vi "MS SQL_Read_Global_Date_v2.vi"(6 "index":i32, 7 "Audit":T1, 8 "error in (no error)":errorcluster, 11 "Ref in":T2={"MS SQL Connection"=refnum, "UDL File"=path "", "Time"="", "DCODE"="", "WIP+1"=0, "MC No?"=0, "POKAYOKE?"=FALSE, "Expected Result"="", "Result [Status]"="", "Clock"=0.0, "RFID"="", "WIP Queue"=refnum, "TS Parameter"={"ProfitCenterCode"="", "LineCode"="", "WorkOrderNumber"="", "Model"="", "Model_with_Prefix"="", "VendorCode"="", "SetParameterDateCode"="", "PokaYoke"=0, "Target"=1, "Live_DateCode"="", "CustomerPartNumber"="", "Hand"="", "Ent_Stamp"=timestamp(0 s since 1904-01-01), "sBarcode"=FALSE, "FCA"=0, "STS_CD"=0.0}, "Data_Queue"=[], "RFID Serial No."=""} {"TS Parameter"."FCA" format="%01d"; "TS Parameter"."Target" min=1 max=100000; "TS Parameter"."PokaYoke" min=0 max=1}) -> (0 "error out":errorcluster, 2 "Date":string[](array[string]), 3 "Ref Out":T2={"MS SQL Connection"=refnum, "UDL File"=path "", "Time"="", "DCODE"="", "WIP+1"=0, "MC No?"=0, "POKAYOKE?"=FALSE, "Expected Result"="", "Result [Status]"="", "Clock"=0.0, "RFID"="", "WIP Queue"=refnum, "TS Parameter"={"ProfitCenterCode"="", "LineCode"="", "WorkOrderNumber"="", "Model"="", "Model_with_Prefix"="", "VendorCode"="", "SetParameterDateCode"="", "PokaYoke"=0, "Target"=1, "Live_DateCode"="", "CustomerPartNumber"="", "Hand"="", "Ent_Stamp"=timestamp(0 s since 1904-01-01), "sBarcode"=FALSE, "FCA"=0, "STS_CD"=0.0}, "Data_Queue"=[], "RFID Serial No."=""} {"TS Parameter"."FCA" format="%01d"; "TS Parameter"."Target" min=1 max=100000; "TS Parameter"."PokaYoke" min=0 max=1})   [LabVIEW 2020]
uses:
  Controls/TD SQL.ctl
  <vilib>/addons/database/Connection.llb/Conn ObjectReference.ctl
  Controls/WIP_State.ctl
  Controls/TS_Parameter.ctl
  <menus>/Controls/Devaseelan Style/ONOFF Small.ctl
  <vilib>/addons/database/Connection.llb/Conn Execute.vi
  <vilib>/addons/database/Recordset.llb/Rec Fetch Recordset Data (R).vi
  <vilib>/addons/database/Recordset.llb/Rec Destroy - Connection.vi
  <userlib>/_OpenG.lib/array/array.llb/Remove Duplicates from 1D Array (String)__ogtk.vi
  <vilib>/addons/database/NI_Database_API.lvlib
panel:
  out "array w/ subset deleted":string[](array[string])
  out "concatenated string":string
  out "result string":string
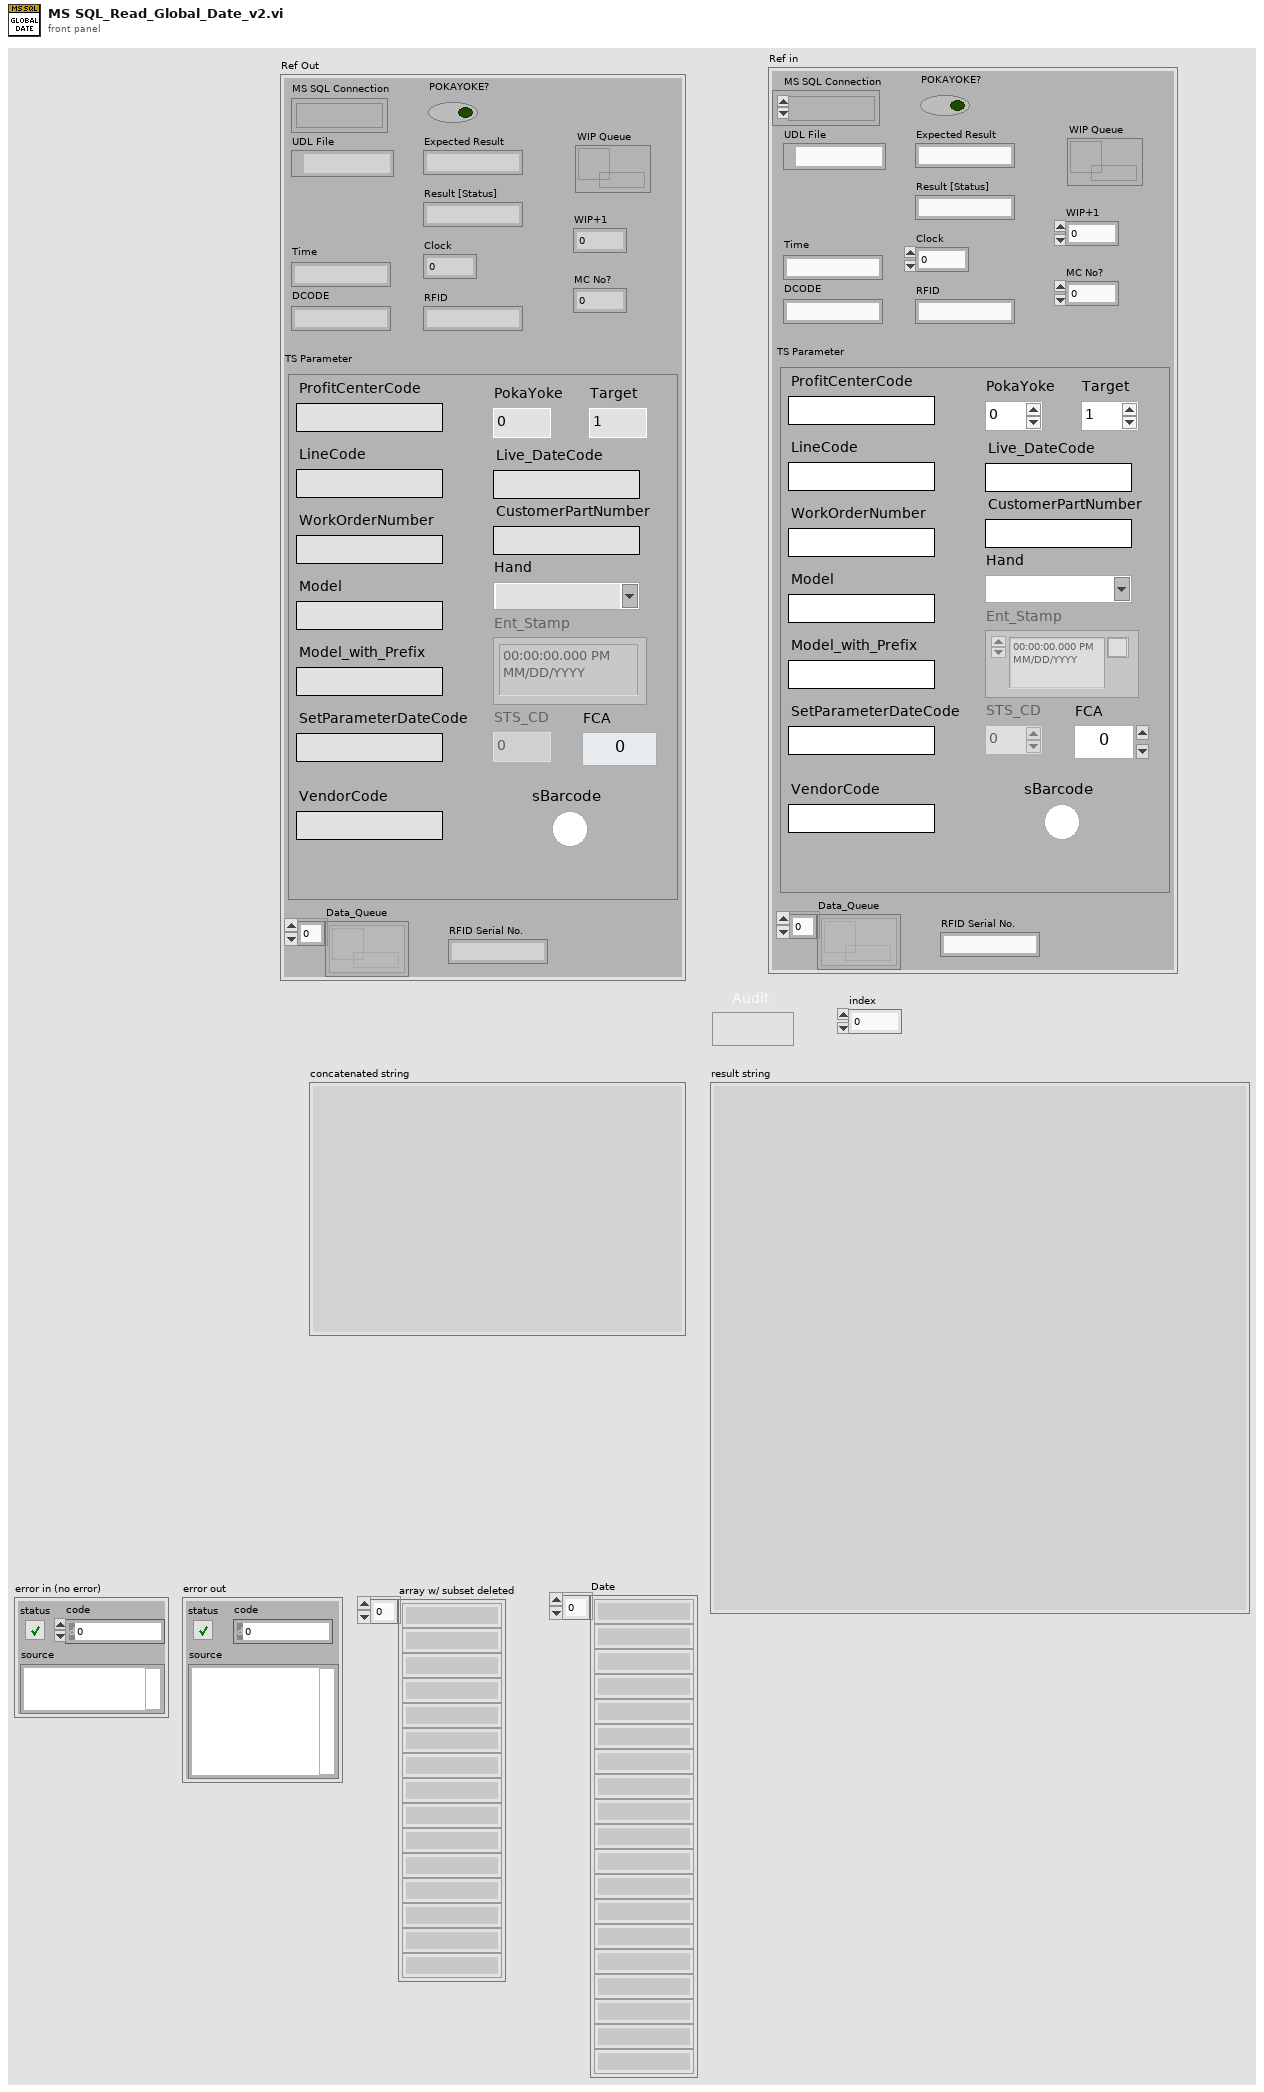
[diagram p1: front panel]
types:
  T1 = typedef "ONOFF Small.ctl" = bool
  T2 = typedef "TD SQL.ctl" = cluster{"MS SQL Connection":T3, "UDL File":path, "Time":string, "DCODE":string, "WIP+1":i64, "MC No?":i32, "POKAYOKE?":bool, "Expected Result":string, "Result [Status]":string, "Clock":dbl, "RFID":string, "WIP Queue":refnum<queue>, "TS Parameter":T4, "Data_Queue":refnum<queue>[], "RFID Serial No.":string}
  T3 = typedef "NI_Database_API.lvlib/Conn ObjectReference.ctl" = refnum<k1>
  T4 = typedef "TS_Parameter.ctl" = cluster{"ProfitCenterCode":string, "LineCode":string, "WorkOrderNumber":string, "Model":string, "Model_with_Prefix":string, "VendorCode":string, "SetParameterDateCode":string, "PokaYoke":i32, "Target":i32, "Live_DateCode":string, "CustomerPartNumber":string, "Hand":string, "Ent_Stamp":timestamp, "sBarcode":bool, "FCA":i32, "STS_CD":dbl}
  T5 = typedef "NI_Database_API.lvlib/Rec ObjectReference.ctl" = refnum<k1>
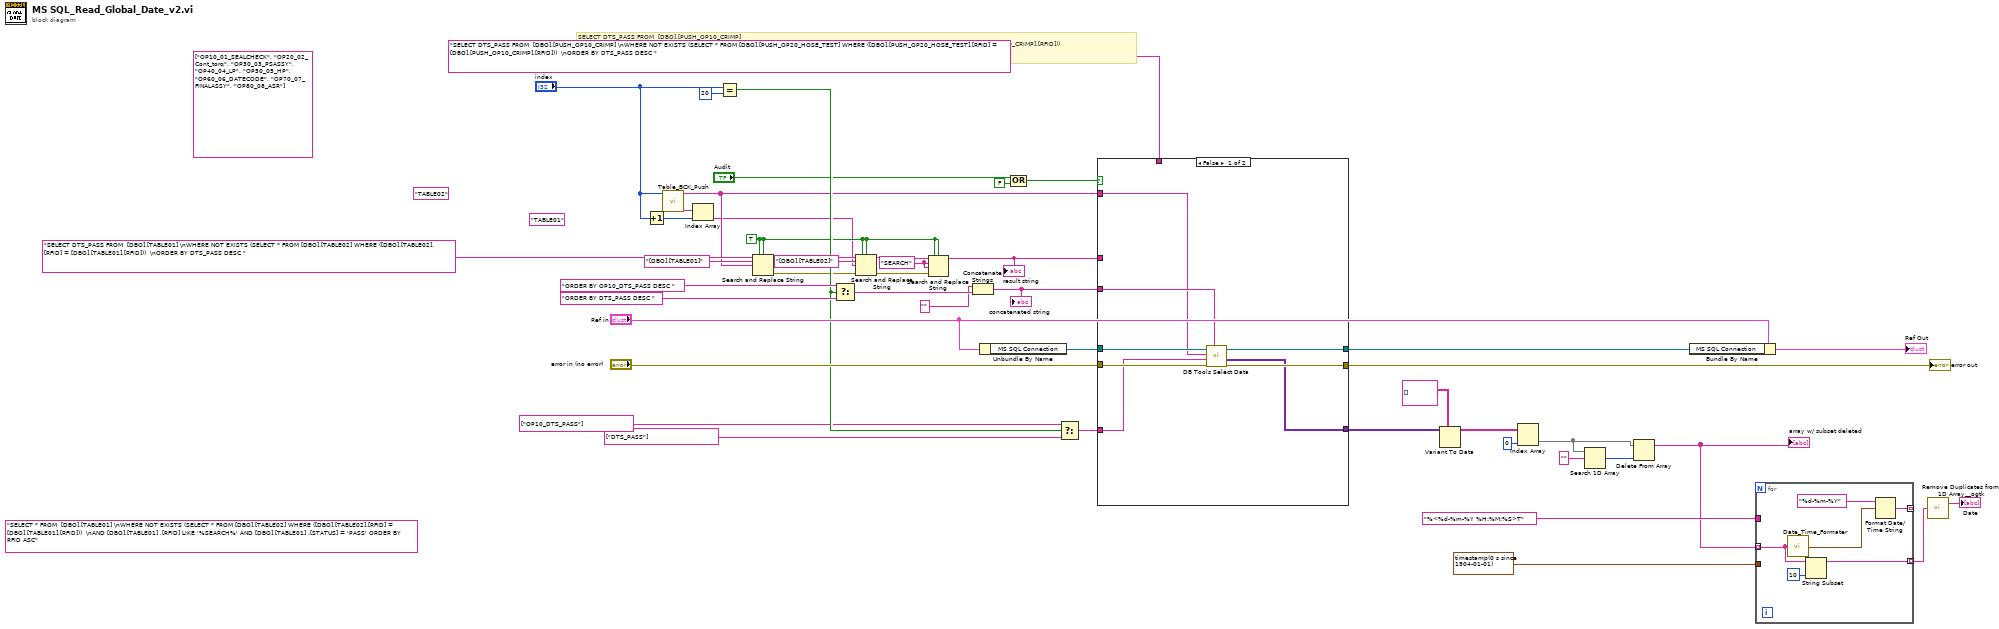
[diagram p0: block diagram]
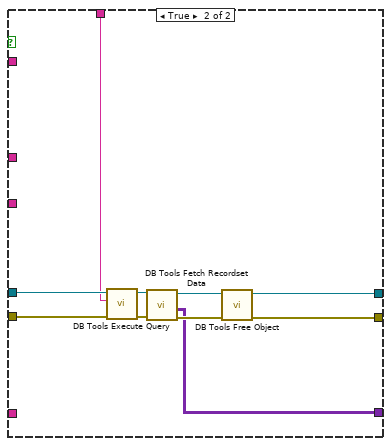
[diagram p2: hidden frame]
diagram:
  (unwired) "TABLE02" ("search string")
  (unwired) "TABLE01" ("search string")
  w8 = "SEARCH" ("search string")
  w18 = TRUE ("replace all? (F)")
  (unwired) "SELECT * FROM  [DBO].[TABLE01] \nWHERE NOT EXISTS (SELECT * FROM [DBO].[TABLE02] WHERE ([DBO].[TABLE02].[RFID] = [DBO].[TABLE01].[RFID]))  \nAND [DBO].[TABLE01] .[RFID] LIKE '%SEARCH%' AND [DBO].[TABLE01] .[STATUS] = 'PASS' ORDER BY RFID ASC"
  (unwired) string[] ["OP10_01_SEALCHECK", "OP20_02_Cont_torq", "OP30_03_PSASSY", "OP40_04_LP", "OP50_05_HP", "OP60_06_DATECODE", "OP70_07_FINALASSY", "OP80_08_ASR"] ("subarray 2")
  # "SELECT DTS_PASS FROM  [DBO].[PUSH_OP10_CRIMP] \nWHERE NOT EXISTS (SELECT * FROM [DBO].[PUSH_OP20_HOSE_TEST] WHERE ([DBO].[PUSH_OP20_HOSE_TEST].[RFID] = [DBO].[PUSH_OP10_CRIMP].[RFID]))  \nORDER BY DTS_PASS DESC"
  n1 = Increment(x="index") -> (x+1=w10:i32)
  n2 = call "Table_BCK_Push.vi"("index"="index") -> ("Tables[]"=w12:string[], "Table Name"=w13:string)  [unwired: 9 in]
  n3 = Index Array(array=w12, index=w10) -> (element=w9:string)
  n4 = Equal?(x="index", y=20) -> (x = y?=w28:bool)
  n5 = Search and Replace String(replace all?=w18, case sensitive?=w18, input string="SELECT DTS_PASS FROM  [DBO].[TABLE01] \nWHERE NOT EXISTS (SELECT * FROM [DBO].[TABLE02] WHERE ([DBO].[TABLE02].[RFID] = [DBO].[TABLE01].[RFID]))  \nORDER BY DTS_PASS DESC ", search string="[DBO].[TABLE01]", replace string=w13) -> (result string=w20:string, error out=w17:errorcluster)  [unwired: 3 in, 2 out]
  n6 = Select(t="ORDER BY OP10_DTS_PASS DESC ", s=w28, f="ORDER BY DTS_PASS DESC ") -> (s? t:f=w29:string)
  n7 = Search and Replace String(replace all?=w18, case sensitive?=w18, input string=w20, search string="[DBO].[TABLE02]", replace string=w9, error in=w17) -> (result string=w19:string, error out=w16:errorcluster)  [unwired: 2 in, 2 out]
  n8 = Search and Replace String(replace all?=w18, case sensitive?=w18, input string=w19, search string=w8, replace string=w8, error in=w16) -> (result string=w14:string)  [unwired: 2 in, 3 out]
  "result string" <- w14
  n9 = Concatenate Strings("" ("time format string (%c)"), w29) -> (w6:string)
  "concatenated string" <- w6
  n10 = Unbundle By Name("Ref in") -> ("MS SQL Connection"=w42:T3)
  n11 = Compound Arithmetic op=OR("Audit", T1 FALSE ("value")) -> (w4:T1)
  n12 = Select(t=string[] ["OP10_DTS_PASS"] ("columns"), s=w28, f=string[] ["DTS_PASS"] ("columns")) -> (s? t:f=w25:string[])
  n13 = case shown="False" w4 {
    tunnel: [w55 w58] -> w46
    tunnel: [w54 w59] -> w45
    tunnel: "error in (no error)" -> [w53 w60]
    tunnel: w42 -> [w52 w61]
    tunnel: w6 -> [w51 _]
    tunnel: w25 -> [w50 _]
    tunnel: w13 -> [w49 _]
    tunnel: [w48 w57] -> w24
    tunnel: w14 -> [_ _]
    tunnel: "SELECT DTS_PASS FROM  [DBO].[PUSH_OP10_CRIMP] \nWHERE NOT EXISTS (SELECT * FROM [DBO].[PUSH_OP20_HOSE_TEST] WHERE ([DBO].[PUSH_OP20_HOSE_TEST].[RFID] = [DBO].[PUSH_OP10_CRIMP].[RFID]))  \nORDER BY DTS_PASS DESC " ("search string") -> [_ w56]
    frame False {
      n14 = call <vilib>:"DB Tools Select Data.vi"("condition"=w51, "error in (no error)"=w53, "columns"=w50, "table"=w49, "connection reference"=w52) -> ("error out"=w55:errorcluster, "data"=w48:variant[][], "connection reference out"=w54:T3)  [unwired: 1 in]
    }
    frame True {
      n15 = call-poly <vilib>:"DB Tools Execute Query.vi"("error in (no error)"=w60, "SQL query"=w56, "connection reference"=w61) -> ("error out"=w62:errorcluster, "recordset reference"=w63:T5)  [unwired: 5 in]
      n16 = call-poly <vilib>:"DB Tools Fetch Recordset Data.vi"("error in (no error)"=w62, "recordset reference"=w63) -> ("error out"=w65:errorcluster, "recordset data"=w57:variant[][], "recordset reference out"=w64:T5)  [unwired: 3 in]
      n17 = call-poly <vilib>:"DB Tools Free Object.vi"("error in (no error)"=w65, "recordset reference"=w64) -> ("error out"=w58:errorcluster, "connection reference"=w59:T3)  [unwired: 8 in]
    }
  }
  "error out" <- w46
  n18 = Variant To Data(type=string[][] [] ("Data"), Variant=w24) -> (data=w41:string[][])  [unwired: 1 in, 1 out]
  n19 = Index Array(array=w41, index (col)=0 ("index (row)")) -> (element=w34:string[])  [unwired: 1 in]
  n20 = Search 1D Array(1D array=w34, element="" ("concatenated string")) -> (index of element=w35:i32)  [unwired: 1 in]
  n21 = Delete From Array(array=w34, index=w35) -> (array with subset deleted=w33:string[])  [unwired: 1 in, 1 out]
  "array w/ subset deleted" <- w33
  n22 = Bundle By Name(cluster="Ref in", "MS SQL Connection"=w45) -> (→"Ref Out":T2)
  n23 = for {
    tunnel: timestamp(0 s since 1904-01-01) ("time stamp") -> [_]
    tunnel: "%<%d-%m-%Y %H:%M:%S>T" ("time format string (%c)") -> [_]
    tunnel: w33 -> [w68] mode=indexing
    tunnel: [w70] -> _ mode=indexing
    tunnel: [w67] -> w1 mode=indexing
    n24 = call "Date_Time_Formater.vi"("Date In"=w68) -> ("Date Out"=w69:timestamp)
    n25 = String Subset(string=w68, length (rest)=10 ("length (rest)")) -> (substring=w67:string)  [unwired: 1 in]
    n26 = Format Date/Time String(time format string (%c)="%d-%m-%Y", seconds (now)=w69) -> (date/time string=w70:string)  [unwired: 1 in]
  }
  n27 = call-poly <userlib>:"Remove Duplicates from 1D Array__ogtk.vi"("Input Array"=w1) -> ("Output Array"=→"Date":string[])  [unwired: 1 out]
